vi "close.vi"(8 "error in (no error)":errorcluster, 11 "file descriptor":i32) -> (0 "error out":errorcluster)   [LabVIEW 2013, in "Linux RT IPC.lvlib" / "Shared Memory.lvlib" / "Shared Memory.lvclass"]
doc: "Wrapper VI for Linux function close()."
uses:
  Shared Memory.lvclass
  Controls/functions.ctl
  <vilib>/NI/NI Linux RT Errno/Linux Errno.lvlib
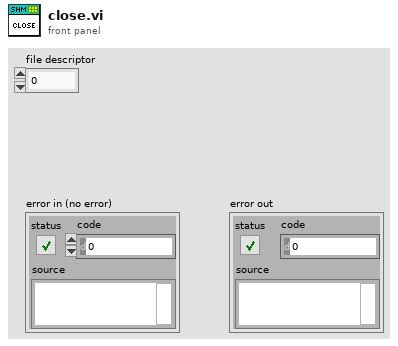
[diagram p1: front panel]
types:
  T1 = typedef "Linux RT IPC.lvlib/Shared Memory.lvlib/Shared Memory.lvclass/functions.ctl" = enum16{"unspecified", "shm_open", "ftruncate", "mmap", "munmap", "close", "shm_unlink", "fstat"}
  T2 = typedef "Linux Errno.lvlib/errno.ctl" = enum16{"NO ERROR", "EPERM", "ENOENT", "ESRCH", "EINTR", "EIO", "ENXIO", "E2BIG", "ENOEXEC", "EBADF", "ECHILD", "EAGAIN", "ENOMEM", "EACCES", "EFAULT", "ENOTBLK", "EBUSY", "EEXIST", "EXDEV", "ENODEV", "ENOTDIR", "EISDIR", "EINVAL", "ENFILE", "EMFILE", "ENOTTY", "ETXTBSY", "EFBIG", "ENOSPC", "ESPIPE", "EROFS", "EMLINK", "EPIPE", "EDOM", "ERANGE", "EDADLK", "ENAMETOOLONG", "ENOLCK", "ENOSYS", "ENOTEMPTY", "ELOOP", "EWOULDBLOCK", "ENOMSG", "EIDRM", "ECHRNG", "EL2NSYNC", "EL3HLT", "EL3RST", "ELNRNG", "EUNATCH", "ENOCSI", "EL2HLT", "EBADE", "EBADR", "EXFULL", "ENOANO", "EBADRQC", "EBADSLT", "EDEADLOCK", "EBFONT", "ENOSTR", "ENODATA", "ETIME", "ENOSR", "ENONET", "ENOPKG", "EREMOTE", "ENOLINK", "EADV", "ESRMNT", "ECOMM", "EPROTO", "EMULTIHOP", "EDOTDOT", "EBADMSG", "EOVERFLOW", "ENOTUNIQ", "EBADFD", "EREMCHG", "ELIBACC", "ELIBBAD", "ELIBSCN", "ELIBMAX", "ELIBEXEC", "ELISEQ", "ERESTART", "ESTRPIPE", "EUSERS", "ENOTSOCK", "EDESTADDRREQ", "EMSGSIZE", "EPROTOTYPE", "ENOPROTOOPT", "EPROTONOSUPPORT", "ESOCKTNOSUPPORT", "EOPNOTSUPP", "EPFNOSUPPORT", "EAFNOSUPPORT", "EADDRINUSE", "EADDRNOTAVAIL", "ENETDOWN", "ENETUNREACH", "ENETRESET", "ECONNABORTED", "ECONNRESET", "ENOBUFS", "EISCONN", "ENOTCONN", "ESHUTDOWN", "ETOOMANYREFS", "ETIMEDOUT", "ECONNREFUSED", "EHOSTDOWN", "EHOSTUNREACH", "EALREADY", "EINPROGRESS", "ESTALE", "EUCLEAN", "ENOTNAM", "ENAVAIL", "EISNAM", "EREMOTEIO", "EDQUOT", "ENOMEDIUM", "EMEDIUMTYPE", "ECANCELED", "ENOKEY", "EKEYEXPIRED", "EKEYREVOKED", "EKEYREJECTED", "EOWNERDEAD", "ENOTRECOVERABLE", "ERFKILL", "EHWPOISON", "UNDEFINED"}
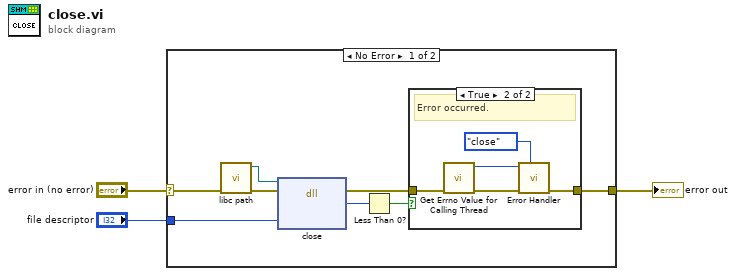
[diagram p0: block diagram]
diagram:
  n1 = case shown="No Error" "error in (no error)" {
    selector: "error in (no error)" -> [w10 w18]
    tunnel: "file descriptor" -> [w11 _]
    tunnel: [w4 w18] -> w2
    frame No Error {
      n2 = call "libc path.vi"("error in (no error)"=w10) -> ("error out"=w9:errorcluster, "path to libc"=w8:path)  [unwired: 9 in]
      n3 = dll-call lib="?" fn="close"(path in=w8, error in=w9, "fd"=w11) -> (error out=w7:errorcluster, "status"=w5:i32)  [unwired: 2 in, 1 out]
      n4 = Less Than 0?(x=w5) -> (x < 0?=w6:bool)
      n5 = case shown="True" w6 {
        tunnel: w7 -> [w12 w17]
        tunnel: [w12 w14] -> w4
        frame False {
          # "No error."
        }
        frame True {
          # "Error occurred."
          n6 = call <vilib>:"Get Errno Value for Calling Thread.vi"("error in (no error)"=w17) -> ("error out"=w15:errorcluster, "errno"=w13:T2)  [unwired: 9 in]
          n7 = call "Error Handler.vi"("function"=functions."close", "error in (no error)"=w15, "errno"=w13) -> ("error out"=w14:errorcluster)  [unwired: 8 in]
        }
      }
    }
    frame Error {
    }
  }
  "error out" <- w2
